vi "CameraTestingProxy_TestPanel.vi"() -> ()   [LabVIEW 2020]
uses:
  CameraTestingApp/ICameraTesting/TypeDef/VideoOptionsInfo.ctl
  ICameraTestingProxy/TypeDef/VideoDataPacket.ctl
  ICameraTestingProxy/TypeDef/VideoFrameData.ctl
  ICameraTestingProxy/TypeDef/ImageType.ctl
  ICameraTestingProxy/TypeDef/Color Model.ctl
  ICameraTestingProxy/TypeDef/Resolution.ctl
  CameraTestingApp/ICameraTesting/TypeDef/CameraInfo.ctl
  Camera/ICamera/ICamera/ICamera.lvclass
  CameraTestingApp/CameraTesting/CameraTesting/CameraTesting.lvclass
  E:/GitHub/Evaluation_Test/Labview/src/CameraTestingApp/ICameraTesting/ICameraTesting/ICameraTesting.lvclass
  CameraTestingProxyAPI/CameraTestingProxyAPI.lvclass
  Camera/CameraI2COUSB/Camera/CameraI2COUSB.lvclass
  E:/GitHub/Evaluation_Test/Labview/src/Camera/ICamera/ICamera/ICamera.lvclass
  Camera/CameraUSB/Camera/Camera.lvclass
  <vilib>/picture/picture.llb/imagedata.ctl
  ICameraTestingProxy/TypeDef/ICameraTestingProxy_typedef.lvlib
  CameraTestingApp/ICameraTesting/TypeDef/ICameraTesting_typedef.lvlib
  E:/GitHub/Evaluation_Test/Labview/src/Camera/CameraI2COUSB/Camera/CameraI2COUSB.lvclass
  E:/GitHub/Evaluation_Test/Labview/src/Camera/CameraUSB/Camera/Camera.lvclass
  C:/Program Files (x86)/National Instruments/LabVIEW 2020/vi.lib/ActorFramework/Actor/Actor.lvclass
  E:/GitHub/Evaluation_Test/Labview/src/CameraTestingApp/CameraTesting/CameraTesting/CameraTesting.lvclass
panel:
  in  "QUIT":bool
  in  "Camera Type":enum32{"I2COUSB", "USB", "Ethernet", "IMAQ"}(tab)
  in  "I2COOUSBParams":T1
  out "Resolution":T2
  in  "Resolution":T2
  in  "Get Res":bool
  in  "Set Res":bool
  out "ImageType":T3
  in  "ImageType":T3
  in  "Get IT":bool
  in  "Set IT":bool
  out "FR":u8
  in  "FR":u8
  in  "Get FR":bool
  in  "Set FR":bool
  out "VideoDataPacket":T5
  out "new picture 2":picture
  in  "Collect":bool
  out "new picture":picture
  out "VideoOptionsInfo":T7
  in  "AcqVideoOptCodes":bool
  in  "Snap":bool
  in  "Stop":bool
  in  "Start":bool
  in  "Disconn":bool
  in  "Conn":bool
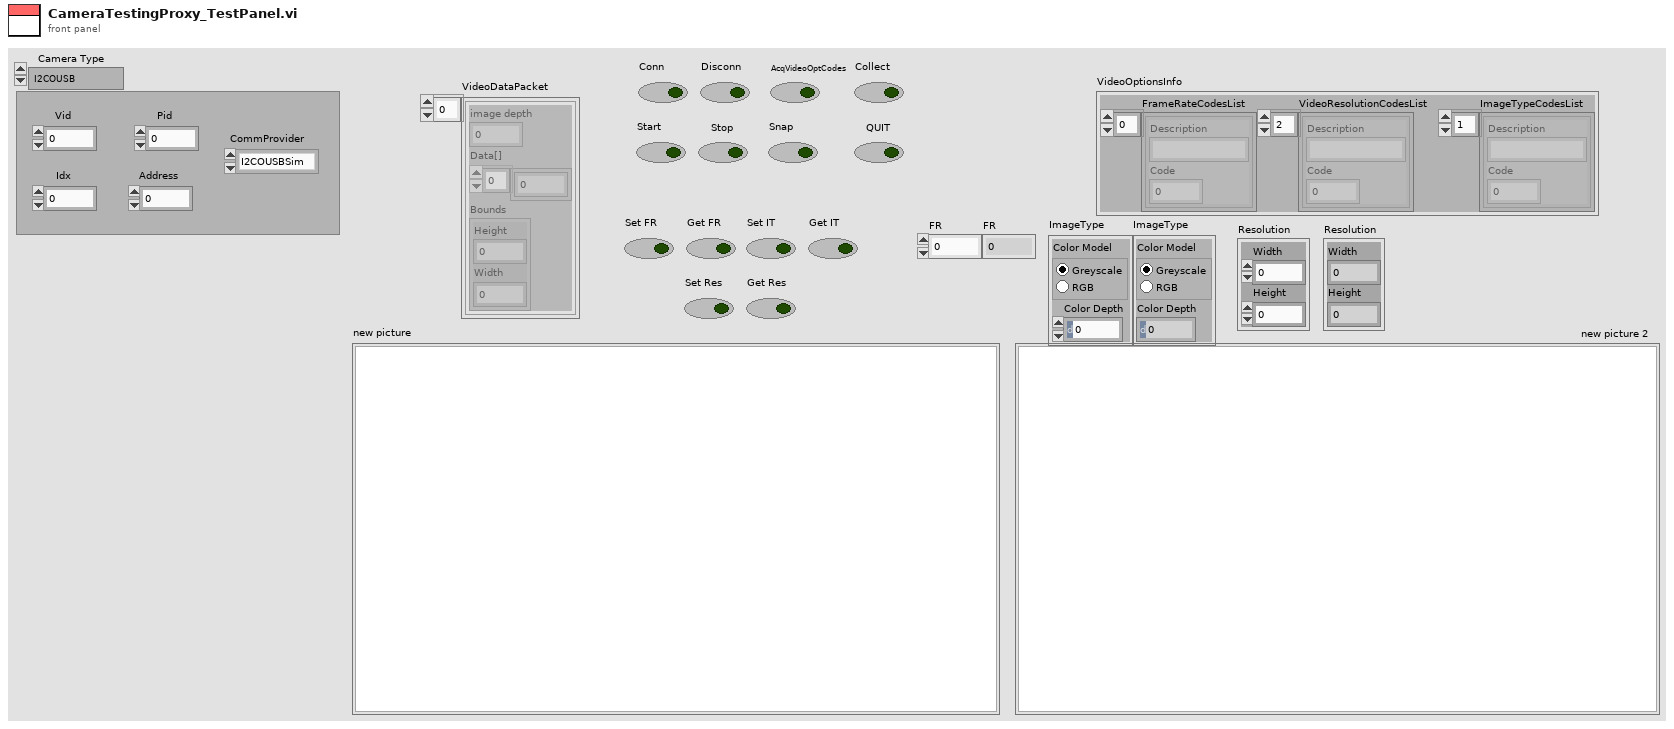
[diagram p1: front panel]
types:
  T1 = cluster{"Vid":u32, "Pid":u32, "Idx":u32, "Address":u32, "CommProvider":enum16{"I2COUSBSim", "ProdType_1", "ProdType_2", "Prod_Type_i", "ProdType_n"}}
  T2 = typedef "ICameraTestingProxy_typedef.lvlib/Resolution.ctl" = cluster{"Width":i16, "Height":i16}
  T3 = typedef "ICameraTestingProxy_typedef.lvlib/ImageType.ctl" = cluster{"Color Model":T4, "Color Depth":u8}
  T4 = typedef "ICameraTestingProxy_typedef.lvlib/Color Model.ctl" = enum32{"Greyscale", "RGB"}
  T5 = typedef "ICameraTestingProxy_typedef.lvlib/VideoDataPacket.ctl" = T6[]
  T6 = typedef "ICameraTestingProxy_typedef.lvlib/VideoFrameData.ctl" = cluster{"image depth":i32, "Data[]":u8[], "Bounds":cluster{"Height":i16, "Width":i16}}
  T7 = typedef "ICameraTesting_typedef.lvlib/VideoOptionsInfo.ctl" = cluster{"FrameRateCodesList":cluster{"Description":string, "Code":u8}[], "VideoResolutionCodesList":cluster{"Description":string, "Code":u8}[], "ImageTypeCodesList":cluster{"Description":string, "Code":u8}[]}
  T8 = typedef "ICameraTesting_typedef.lvlib/CameraInfo.ctl" = cluster{"ICamera ":refnum<class "ICamera.lvclass">, "Connection String":string}
  T9 = enum16{"I2COUSBSim", "ProdType_1", "ProdType_2", "Prod_Type_i", "ProdType_n"}
  T10 = typedef "imagedata.ctl" = cluster{"image type":i32, "image depth":i32, "image":u8[], "mask":u8[], "colors":u32[], "Rectangle":cluster{"left":i16, "top":i16, "right":i16, "bottom":i16}}
  T11 = typedef "ICameraTestingProxy_typedef.lvlib/SnapData.ctl" = cluster{"image depth":i32, "PixelData":u8[], "Resolution":T2}
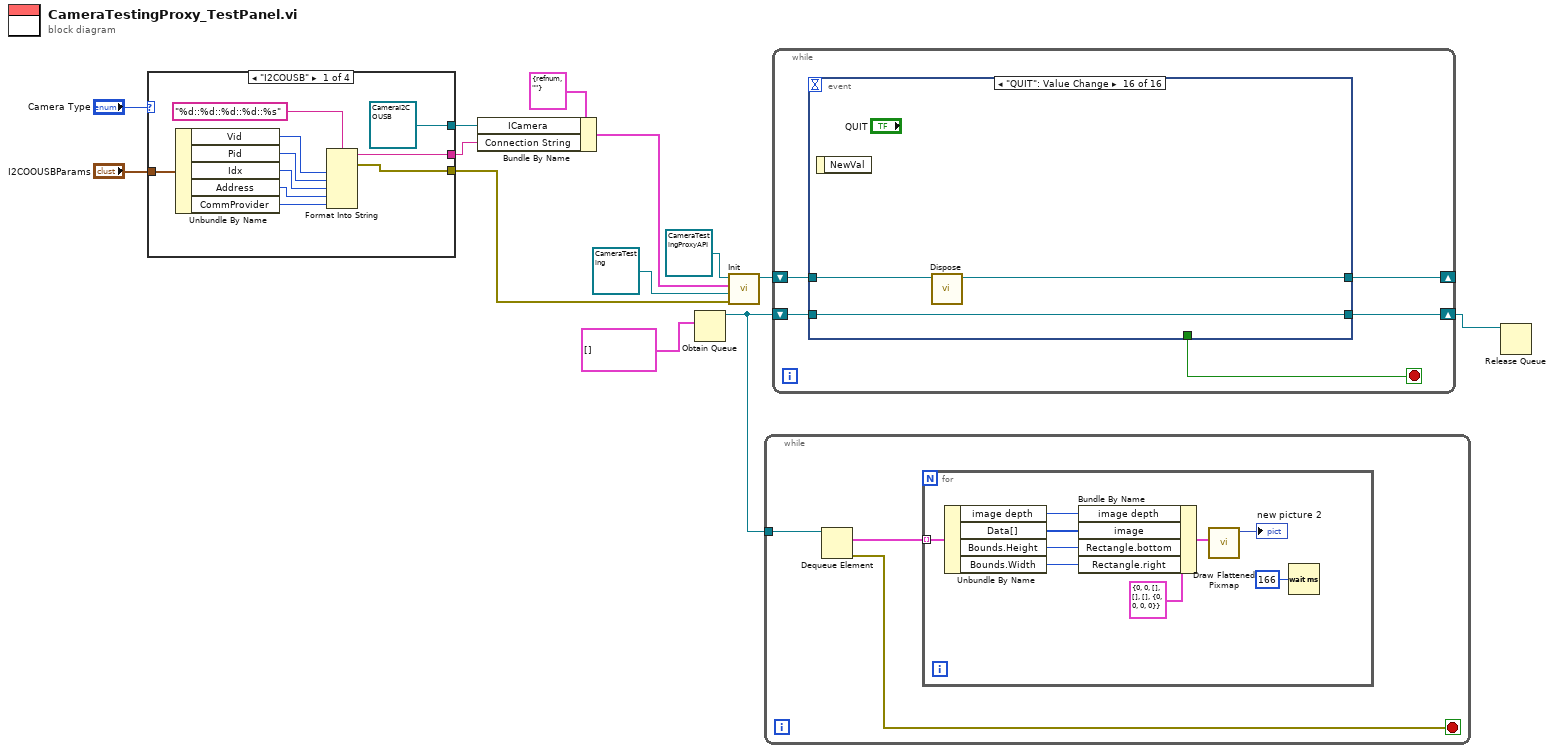
[diagram p0: block diagram]
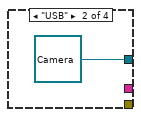
[diagram p2: hidden frame]
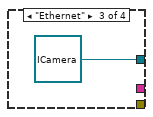
[diagram p3: hidden frame]
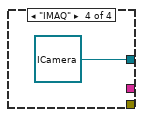
[diagram p4: hidden frame]
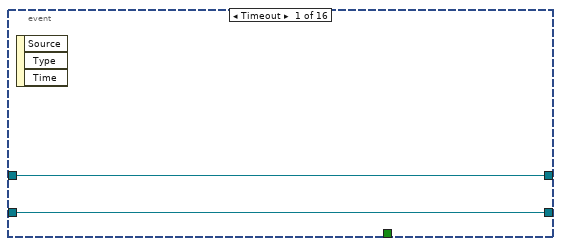
[diagram p5: hidden frame]
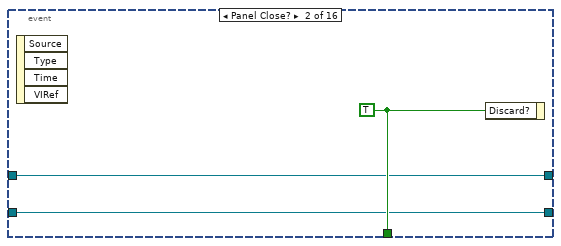
[diagram p6: hidden frame]
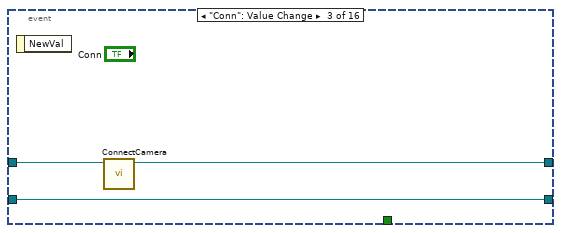
[diagram p7: hidden frame]
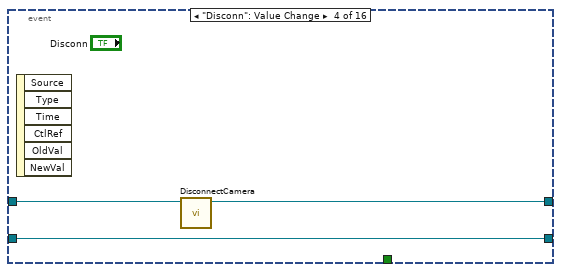
[diagram p8: hidden frame]
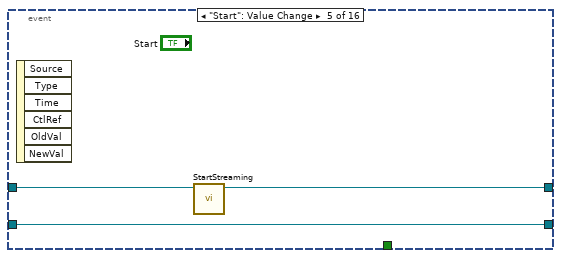
[diagram p9: hidden frame]
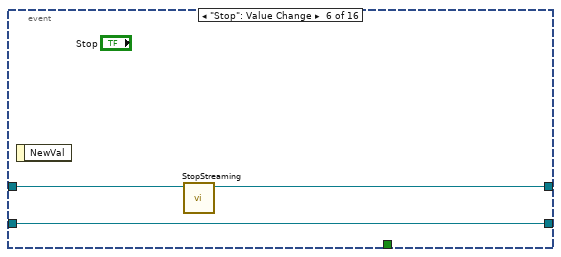
[diagram p10: hidden frame]
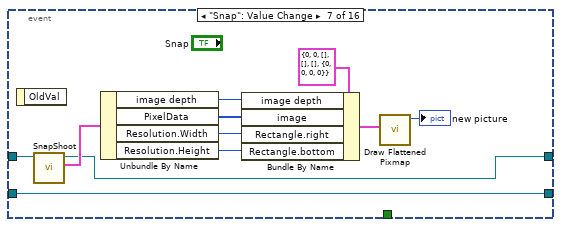
[diagram p11: hidden frame]
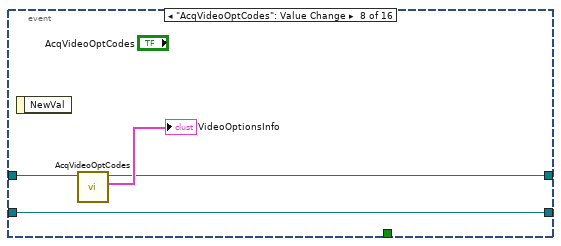
[diagram p12: hidden frame]
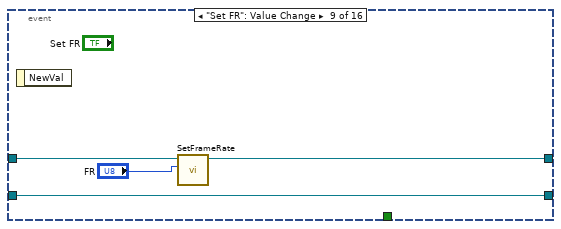
[diagram p13: hidden frame]
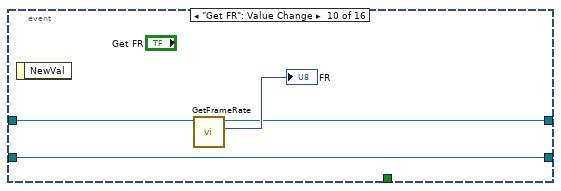
[diagram p14: hidden frame]
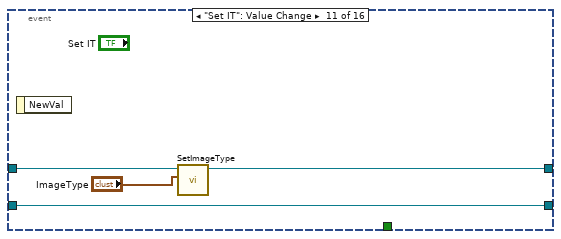
[diagram p15: hidden frame]
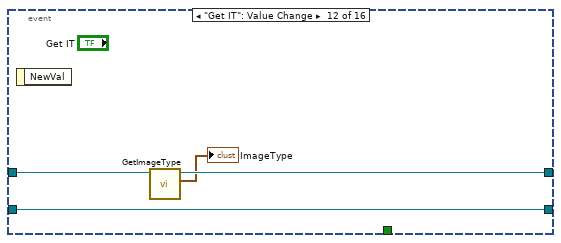
[diagram p16: hidden frame]
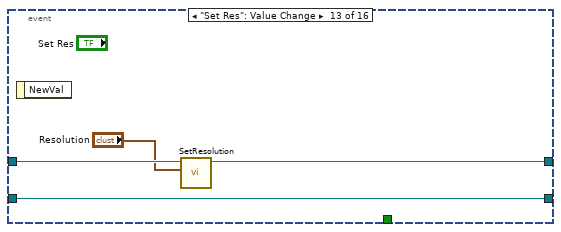
[diagram p17: hidden frame]
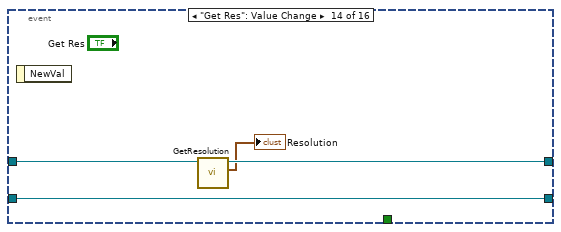
[diagram p18: hidden frame]
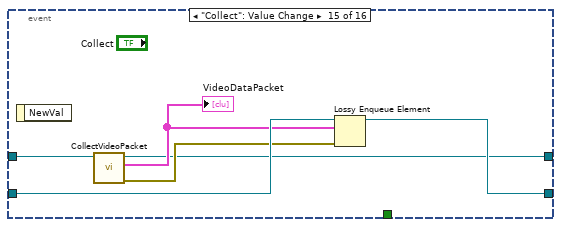
[diagram p19: hidden frame]
diagram:
  n1 = case shown="\"I2COUSB\"" "Camera Type" {
    tunnel: "I2COOUSBParams" -> [w22 _ _ _]
    tunnel: [refnum<class "CameraI2COUSB.lvclass"> refnum ("CameraDemo in") refnum<class "Camera.lvclass"> refnum ("CameraUSB.lvlib:Camera.lvclass") refnum<class "ICamera.lvclass"> refnum ("ICamera.lvlib:ICamera.lvclass") refnum<class "ICamera.lvclass"> refnum ("ICamera.lvlib:ICamera.lvclass")] -> w7
    tunnel: [w15 _ _ _] -> w6
    tunnel: [w14 _ _ _] -> w4
    frame "I2COUSB" {
      n2 = Unbundle By Name(w22) -> ("Vid"=w21:u32, "Pid"=w20:u32, "Idx"=w19:u32, "Address"=w18:u32, "CommProvider"=w17:T9)
      n3 = Format Into String(format string="%d::%d::%d::%d::%s", w21, w20, w19, w18, w17) -> (resulting string=w15:string, error out=w14:errorcluster)  [unwired: 2 in]
    }
    frame "USB" {
    }
    frame "Ethernet" {
    }
    frame "IMAQ" {
    }
  }
  n4 = Bundle By Name(cluster=T8 {"ICamera "=refnum, "Connection String"=""} ("CameraInfo"), "ICamera"=w7, "Connection String"=w6) -> (w2:T8)
  n5 = Obtain Queue(element data type=T5 [] ("VideoDataPacket")) -> (queue out=w12:refnum<queue>)  [unwired: 4 in, 2 out]
  n6 = call-dynamic "Init.vi"("error in (no error)"=w4, "ICameraTesting"=refnum<class "CameraTesting.lvclass"> refnum ("CameraTesting.lvlib:CameraTesting.lvclass"), "CameraInfo"=w2, "CameraTestingProxy"=refnum<class "CameraTestingProxyAPI.lvclass"> refnum ("CameraTestingProxy.lvlib:CameraTestingProxyAPI.lvclass")) -> ("CameraTestingProxy"=w5:refnum<class "CameraTestingProxyAPI.lvclass">)  [unwired: 6 in, 1 out]
  n7 = while {
    tunnel: w12 -> [w29]
    stop <- w27 stop-if-true
    n8 = Dequeue Element(queue=w29) -> (element=w28:T5, error out=w27:errorcluster)  [unwired: 2 in, 2 out]
    n9 = for {
      tunnel: w28 -> [w35] mode=indexing
      n10 = Unbundle By Name(w35) -> ("image depth"=w34:i32, "Data[]"=w33:u8[], "Bounds.Height"=w31:i16, "Bounds.Width"=w32:i16)
      n11 = Bundle By Name(cluster=T10 {"image type"=0, "image depth"=0, "image"=[], "mask"=[], "colors"=[], "Rectangle"={"left"=0, "top"=0, "right"=0, "bottom"=0}} ("image data"), "image depth"=w34, "image"=w33, "Rectangle.bottom"=w31, "Rectangle.right"=w32) -> (w36:T10)
      n12 = call <vilib>:"Draw Flattened Pixmap.vi"("image data"=w36) -> ("new picture"=→"new picture 2":picture)  [unwired: 8 in]
      n13 = Wait (ms)(milliseconds to wait=u32 166) -> ()  [unwired: 1 out]
    }
  }
  n14 = while {
    shift-right: [w40] -> w11
    shift-left: w12 -> [w41]
    shift-right: [w39] -> _
    shift-left: w5 -> [w43]
    stop <- w42 stop-if-true
    n15 = event shown="[15] \"QUIT\": Value Change" {
      selector: _ -> [_ _ _ _ _ _ _ _ _ _ _ _ _ _ _ _]
      dyn-events: _ -> [_ _ _ _ _ _ _ _ _ _ _ _ _ _ _ _]
      timeout: _ -> [_ _ _ _ _ _ _ _ _ _ _ _ _ _ _ _]
      tunnel: w43 -> [w44 w46 w51 w54 w57 w60 w71 w75 w78 w82 w85 w89 w94 w98 w105 w107]
      tunnel: [_ w48 _ _ _ _ _ _ _ _ _ _ _ _ _ _] -> w42
      tunnel: w41 -> [w45 w47 w50 w53 w56 w59 w62 w73 w79 w83 w87 w91 w95 w99 w104 w108]
      tunnel: [w45 w47 w50 w53 w56 w59 w62 w73 w79 w83 w87 w91 w95 w99 w102 w108] -> w40
      tunnel: [w44 w46 w49 w52 w55 w58 w61 w72 w76 w80 w86 w90 w93 w97 w100 w106] -> w39
      event Timeout {
        n16 = event-data() -> ()  [unwired: 1 in, 3 out]
      }
      event Panel Close? {
        w48 = TRUE ("Discard?")
        n17 = event-data() -> ()  [unwired: 1 in, 4 out]
        n18 = event-data("Discard?"=w48) -> ()  [unwired: 1 in, 1 out]
      }
      event "Conn": Value Change {
        n19 = event-data() -> ()  [unwired: 1 in, 1 out]
        n20 = call-dynamic "ConnectCamera.vi"("CameraTestingProxy in"=w51) -> ("CameraTestingProxy out"=w49:refnum<class "CameraTestingProxyAPI.lvclass">)  [unwired: 9 in, 1 out]
      }
      event "Disconn": Value Change {
        n21 = event-data() -> ()  [unwired: 1 in, 6 out]
        n22 = call-dynamic "DisconnectCamera.vi"("CameraTestingProxy in"=w54) -> ("CameraTestingProxy out"=w52:refnum<class "CameraTestingProxyAPI.lvclass">)  [unwired: 9 in, 1 out]
      }
      event "Start": Value Change {
        n23 = event-data() -> ()  [unwired: 1 in, 6 out]
        n24 = call-dynamic "StartStreaming.vi"("CameraTestingProxy in"=w57) -> ("CameraTestingProxy out"=w55:refnum<class "CameraTestingProxyAPI.lvclass">)  [unwired: 9 in, 1 out]
      }
      event "Stop": Value Change {
        n25 = event-data() -> ()  [unwired: 1 in, 1 out]
        n26 = call-dynamic "StopStreaming.vi"("CameraTestingProxy in"=w60) -> ("CameraTestingProxy out"=w58:refnum<class "CameraTestingProxyAPI.lvclass">)  [unwired: 9 in, 1 out]
      }
      event "Snap": Value Change {
        n27 = event-data() -> ()  [unwired: 1 in, 1 out]
        n28 = call-dynamic "SnapShoot.vi"("CameraTestingProxy in"=w71) -> ("SnapData"=w68:T11, "CameraTestingProxy out"=w61:refnum<class "CameraTestingProxyAPI.lvclass">)  [unwired: 8 in, 1 out]
        n29 = Unbundle By Name(w68) -> ("image depth"=w67:i32, "PixelData"=w66:u8[], "Resolution.Width"=w65:i16, "Resolution.Height"=w64:i16)
        n30 = Bundle By Name(cluster=T10 {"image type"=0, "image depth"=0, "image"=[], "mask"=[], "colors"=[], "Rectangle"={"left"=0, "top"=0, "right"=0, "bottom"=0}} ("image data"), "image depth"=w67, "image"=w66, "Rectangle.right"=w65, "Rectangle.bottom"=w64) -> (w70:T10)
        n31 = call <vilib>:"Draw Flattened Pixmap.vi"("image data"=w70) -> ("new picture"=→"new picture":picture)  [unwired: 8 in]
      }
      event "AcqVideoOptCodes": Value Change {
        n32 = event-data() -> ()  [unwired: 1 in, 1 out]
        n33 = call-dynamic "AcqVideoOptCodes.vi"("CameraTestingProxyAPI in"=w75) -> ("VideoOptionsInfo"=→"VideoOptionsInfo":T7, "CameraTestingProxyAPI out"=w72:refnum<class "CameraTestingProxyAPI.lvclass">)  [unwired: 8 in, 1 out]
      }
      event "Set FR": Value Change {
        n34 = event-data() -> ()  [unwired: 1 in, 1 out]
        n35 = call-dynamic "SetFrameRate.vi"("Frame Rate"="FR", "CameraTestingProxyAPI in"=w78) -> ("CameraTestingProxyAPI out"=w76:refnum<class "CameraTestingProxyAPI.lvclass">)  [unwired: 8 in, 1 out]
      }
      event "Get FR": Value Change {
        n36 = event-data() -> ()  [unwired: 1 in, 1 out]
        n37 = call-dynamic "GetFrameRate.vi"("CameraTestingProxyAPI in"=w82) -> ("Frame Rate"=→"FR":u8, "CameraTestingProxyAPI out"=w80:refnum<class "CameraTestingProxyAPI.lvclass">)  [unwired: 8 in, 1 out]
      }
      event "Set IT": Value Change {
        n38 = event-data() -> ()  [unwired: 1 in, 1 out]
        n39 = call-dynamic "SetImageType.vi"("ImageType"="ImageType", "CameraTestingProxyAPI in"=w85) -> ("CameraTestingProxyAPI out"=w86:refnum<class "CameraTestingProxyAPI.lvclass">)  [unwired: 8 in, 1 out]
      }
      event "Get IT": Value Change {
        n40 = event-data() -> ()  [unwired: 1 in, 1 out]
        n41 = call-dynamic "GetImageType.vi"("CameraTestingProxyAPI in"=w89) -> ("ImageType"=→"ImageType":T3, "CameraTestingProxyAPI out"=w90:refnum<class "CameraTestingProxyAPI.lvclass">)  [unwired: 8 in, 1 out]
      }
      event "Set Res": Value Change {
        n42 = event-data() -> ()  [unwired: 1 in, 1 out]
        n43 = call-dynamic "SetResolution.vi"("Resolution"="Resolution", "CameraTestingProxyAPI in"=w94) -> ("CameraTestingProxyAPI out"=w93:refnum<class "CameraTestingProxyAPI.lvclass">)  [unwired: 8 in, 1 out]
      }
      event "Get Res": Value Change {
        n44 = event-data() -> ()  [unwired: 1 in, 1 out]
        n45 = call-dynamic "GetResolution.vi"("CameraTestingProxyAPI in"=w98) -> ("Resolution"=→"Resolution":T2, "CameraTestingProxyAPI out"=w97:refnum<class "CameraTestingProxyAPI.lvclass">)  [unwired: 7 in, 2 out]
      }
      event "Collect": Value Change {
        n46 = event-data() -> ()  [unwired: 1 in, 1 out]
        n47 = call-dynamic "CollectVideoPacket.vi"("CameraTestingProxyAPI in"=w105) -> ("error out"=w101:errorcluster, "VideoDataPacket"=w103:T5, "CameraTestingProxyAPI out"=w100:refnum<class "CameraTestingProxyAPI.lvclass">)  [unwired: 8 in]
        "VideoDataPacket" <- w103
        n48 = Lossy Enqueue Element(queue=w104, element=w103, error in (no error)=w101) -> (queue out=w102:refnum<queue>)  [unwired: 3 out]
      }
      event "QUIT": Value Change {
        n49 = event-data() -> ()  [unwired: 1 in, 1 out]
        n50 = call-dynamic "Dispose.vi"("CameraTestingProxyAPI in"=w107) -> ("CameraTestingProxyAPI out"=w106:refnum<class "CameraTestingProxyAPI.lvclass">)  [unwired: 9 in, 1 out]
      }
    }
  }
  n51 = Release Queue(queue=w11) -> ()  [unwired: 2 in, 3 out]
